vi "Create.vi"(7 "Frequency (kHz)":dbl=12.0 format="%#_13g") -> (8 "Tone":refnum<class "Tone.lvclass">)   [LabVIEW 2020, in "Tone.lvclass"]
uses:
  Tone.lvclass
  Tone.lvclass/Tone.ctl
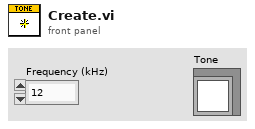
[diagram p1: front panel]
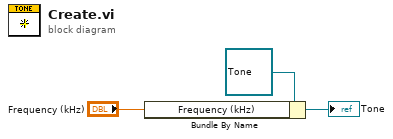
[diagram p0: block diagram]
diagram:
  n1 = Bundle By Name(cluster=refnum<class "Tone.lvclass"> refnum ("Tone"), "Frequency (kHz)"="Frequency (kHz)") -> (→"Tone":refnum<class "Tone.lvclass">)
